vi "Read nbrStepsInProfile.vi"(11 "TestMonitor in":refnum<class "TestMonitor.lvclass">) -> (2 "nbrStepsInProfile":u32 min=1, 3 "TestMonitor out":refnum<class "TestMonitor.lvclass">)   [LabVIEW 2013, in "TestMonitor.lvclass"]
uses:
  TestMonitor.lvclass
  TestMonitor.lvclass/TestMonitor.ctl
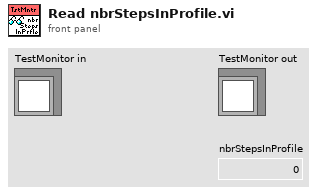
[diagram p1: front panel]
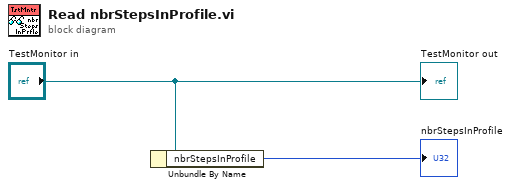
[diagram p0: block diagram]
diagram:
  n1 = Unbundle By Name("TestMonitor in") -> ("nbrStepsInProfile"=→"nbrStepsInProfile":u32)
  "TestMonitor out" <- "TestMonitor in"
